vi "Contour Line_Find Candidate Edges (point).vi"(11 "edge":T2) -> (3 "Candidate Edges":T1(array[cluster]))   [LabVIEW 2020, in "NI_AAL_Geometry.lvlib"]
uses:
  <vilib>/Analysis/NI_AAL_Geometry.lvlib
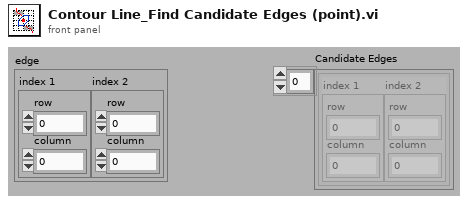
[diagram p1: front panel]
types:
  T1 = cluster{"index 1":cluster{"row":i32, "column":i32}, "index 2":cluster{"row":i32, "column":i32}}[]
  T2 = cluster{"index 1":cluster{"row":i32, "column":i32}, "index 2":cluster{"row":i32, "column":i32}}
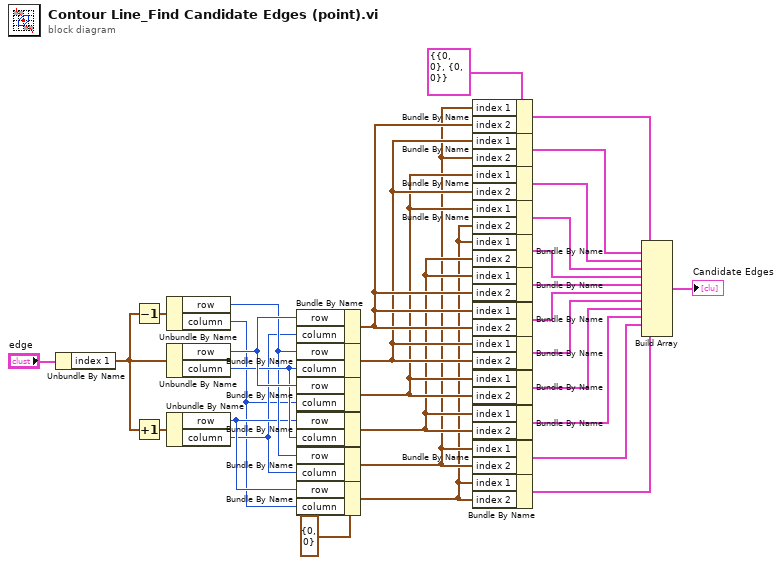
[diagram p0: block diagram]
diagram:
  w18 = cluster{"row":i32, "column":i32} {"row"=0, "column"=0} ("index 2")
  w6 = T2 {"index 1"={"row"=0, "column"=0}, "index 2"={"row"=0, "column"=0}} ("edge")
  n1 = Unbundle By Name("edge") -> ("index 1"=w21:cluster{"row":i32, "column":i32})
  n2 = Decrement(x=w21) -> (x-1=w22:cluster{"row":i32, "column":i32})
  n3 = Increment(x=w21) -> (x+1=w23:cluster{"row":i32, "column":i32})
  n4 = Unbundle By Name(w22) -> ("row"=w17:i32, "column"=w14:i32)
  n5 = Unbundle By Name(w21) -> ("row"=w20:i32, "column"=w19:i32)
  n6 = Unbundle By Name(w23) -> ("row"=w16:i32, "column"=w15:i32)
  n7 = Bundle By Name(cluster=w18, "row"=w20, "column"=w15) -> (w13:cluster{"row":i32, "column":i32})
  n8 = Bundle By Name(cluster=w18, "row"=w17, "column"=w19) -> (w12:cluster{"row":i32, "column":i32})
  n9 = Bundle By Name(cluster=w18, "row"=w20, "column"=w14) -> (w11:cluster{"row":i32, "column":i32})
  n10 = Bundle By Name(cluster=w18, "row"=w16, "column"=w19) -> (w10:cluster{"row":i32, "column":i32})
  n11 = Bundle By Name(cluster=w18, "row"=w17, "column"=w15) -> (w9:cluster{"row":i32, "column":i32})
  n12 = Bundle By Name(cluster=w18, "row"=w16, "column"=w14) -> (w8:cluster{"row":i32, "column":i32})
  n13 = Bundle By Name(cluster=w6, "index 1"=w9, "index 2"=w13) -> (w30:T2)
  n14 = Bundle By Name(cluster=w6, "index 1"=w12, "index 2"=w9) -> (w29:T2)
  n15 = Bundle By Name(cluster=w6, "index 1"=w11, "index 2"=w12) -> (w28:T2)
  n16 = Bundle By Name(cluster=w6, "index 1"=w11, "index 2"=w8) -> (w27:T2)
  n17 = Bundle By Name(cluster=w6, "index 1"=w8, "index 2"=w10) -> (w26:T2)
  n18 = Bundle By Name(cluster=w6, "index 1"=w10, "index 2"=w13) -> (w25:T2)
  n19 = Bundle By Name(cluster=w6, "index 1"=w13, "index 2"=w13) -> (w7:T2)
  n20 = Bundle By Name(cluster=w6, "index 1"=w12, "index 2"=w12) -> (w5:T2)
  n21 = Bundle By Name(cluster=w6, "index 1"=w11, "index 2"=w11) -> (w4:T2)
  n22 = Bundle By Name(cluster=w6, "index 1"=w10, "index 2"=w10) -> (w3:T2)
  n23 = Bundle By Name(cluster=w6, "index 1"=w9, "index 2"=w9) -> (w2:T2)
  n24 = Bundle By Name(cluster=w6, "index 1"=w8, "index 2"=w8) -> (w1:T2)
  n25 = Build Array(w30, w29, w28, w27, w26, w25, w7, w5, w4, w3, w2, w1) -> (→"Candidate Edges":T1)
